vi "TrALEX_GRN.vi"(0 "Analog Amplitude":dbl=1.0 format="%0.2p", 1 "Repetition Frequency":dbl=2.0 format="%.6f") -> ()   [LabVIEW 2011]
uses:
  <vilib>/DAQmx/write.llb/DAQmx Write (Analog Wfm 1Chan NSamp).vi
  <vilib>/DAQmx/create/channels.llb/DAQmx Create Channel (AO-Voltage-Basic).vi
  <vilib>/DAQmx/configure/timing.llb/DAQmx Timing (Sample Clock).vi
  <vilib>/DAQmx/create/channels.llb/DAQmx Create Channel (CO-Pulse Generation-Frequency).vi
  <vilib>/DAQmx/configure/events/hardwareSignals.llb/DAQmx Export Signal (Most Signals).vi
  <vilib>/DAQmx/configure/trigger.llb/DAQmx Start Trigger (Digital Edge).vi
  <vilib>/DAQmx/configure/timing.llb/DAQmx Timing (Implicit).vi
  <vilib>/DAQmx/miscellaneous.llb/DAQmx Fill In Error Info.vi
  <vilib>/measure/NI_MABase.lvlib
panel:
  in  "Three Colour Duty Cycle":dbl=0.3333333333333333 format="%.6f"
  in  "Stop Button":bool
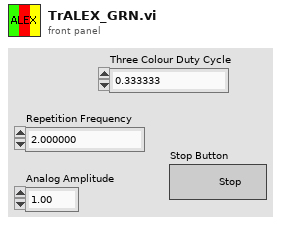
[diagram p1: front panel]
types:
  T1 = enum16{"Sine Wave", "Triangle Wave", "Square Wave", "Sawtooth Wave"}
  T2 = cluster{"Ao0 Sample Clock Rate":dbl, "Ao0 Sample Clock Rate":dbl}
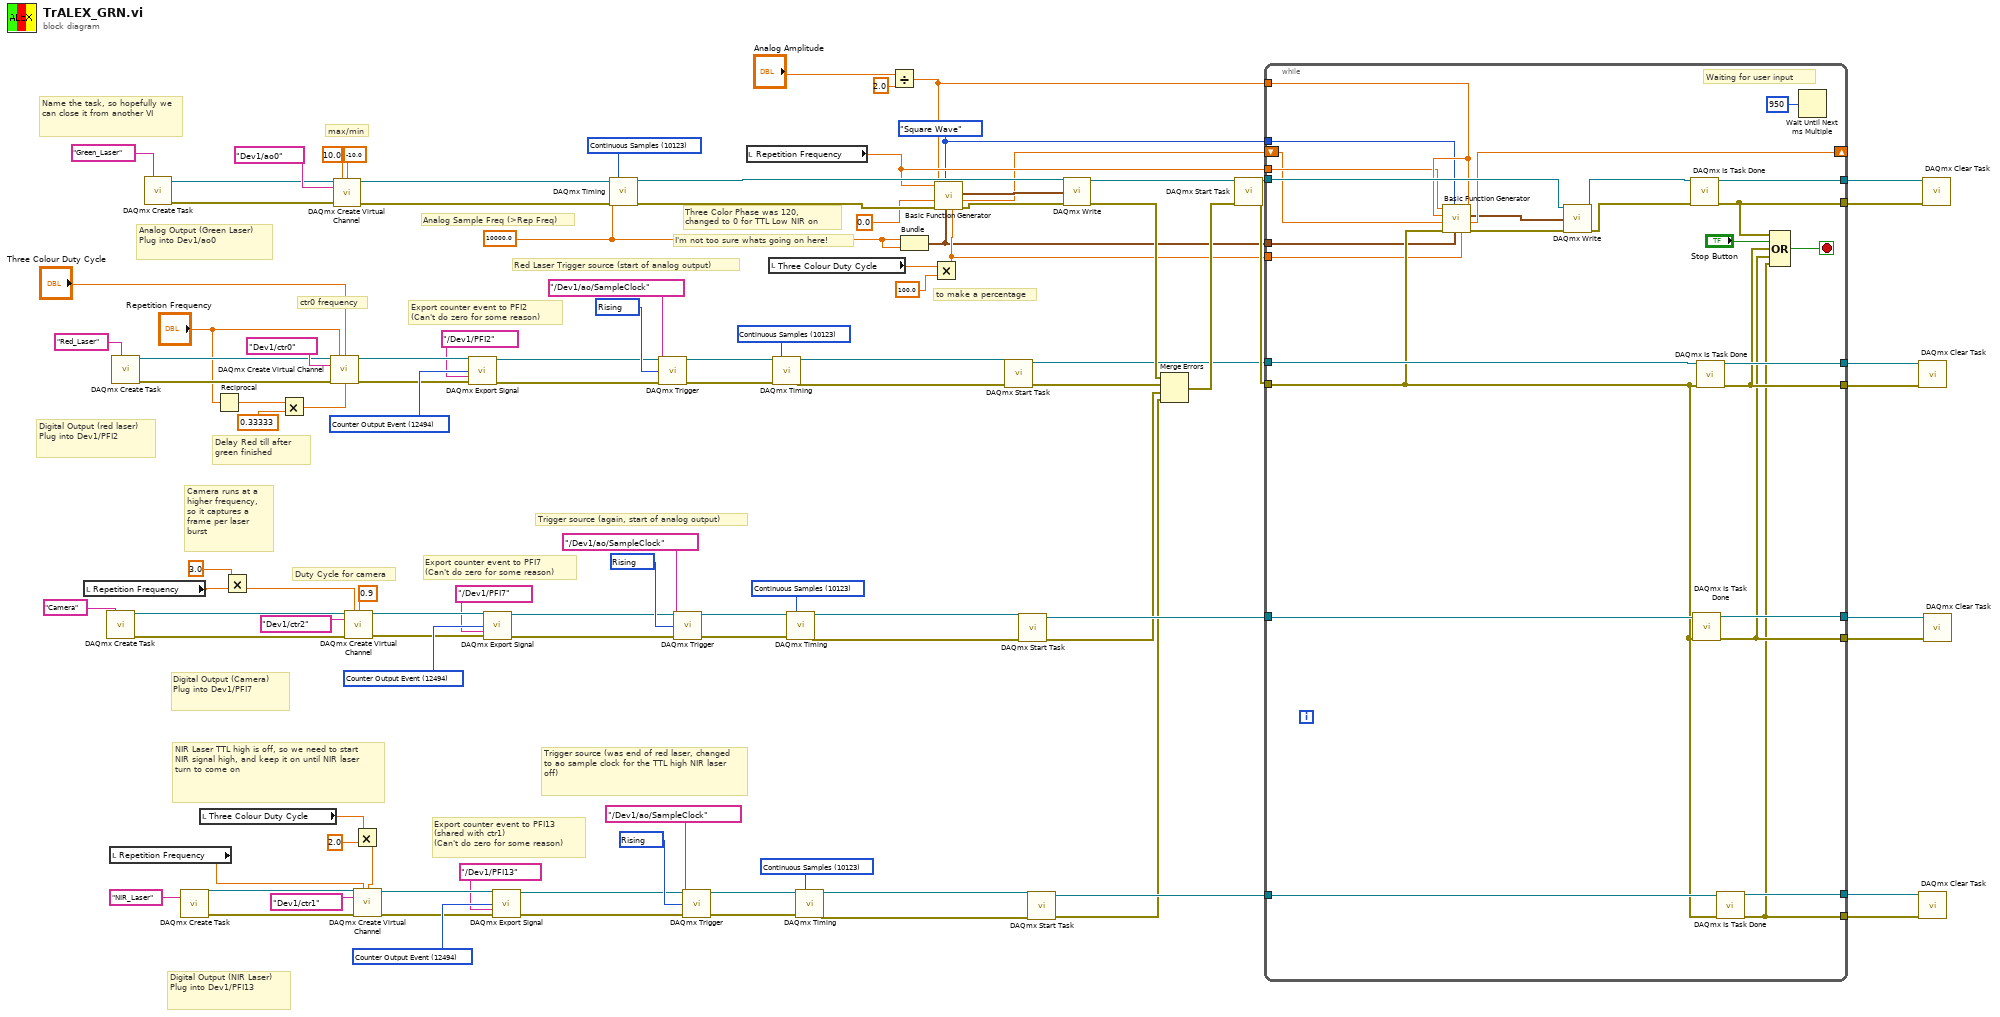
[diagram p0: block diagram]
diagram:
  w41 = 10280 items=["Rising"=10280, "Falling"=10171] ("edge")
  w44 = 10123 items=["Finite Samples"=10178, "Continuous Samples"=10123, "Hardware Timed Single Point"=12522] ("sample mode")
  w46 = 12494 items=["AI Convert Clock"=12484, "10MHz Reference Clock"=12536, "20MHz Timebase Clock"=12486, "Sample Clock"=12487, "Advance Trigger"=12488, "Reference Trigger"=12490, "Start Trigger"=12491, "Advance Complete Event"=12492, "AI Hold Complete Event"=12493, "Counter Output Event"=12494, "Change Detection Event"=12511, "Watchdog Timer Expired Event"=12512] ("signal")
  w64 = 10280 items=["Rising"=10280, "Falling"=10171] ("edge")
  w67 = 10123 items=["Finite Samples"=10178, "Continuous Samples"=10123, "Hardware Timed Single Point"=12522] ("sample mode")
  w69 = 12494 items=["AI Convert Clock"=12484, "10MHz Reference Clock"=12536, "20MHz Timebase Clock"=12486, "Sample Clock"=12487, "Advance Trigger"=12488, "Reference Trigger"=12490, "Start Trigger"=12491, "Advance Complete Event"=12492, "AI Hold Complete Event"=12493, "Counter Output Event"=12494, "Change Detection Event"=12511, "Watchdog Timer Expired Event"=12512] ("signal")
  w75 = 10123 items=["Finite Samples"=10178, "Continuous Samples"=10123, "Hardware Timed Single Point"=12522] ("sample mode")
  w7 = T1."Square Wave" ("signal type")
  w95 = 10280 items=["Rising"=10280, "Falling"=10171] ("edge")
  w100 = 10123 items=["Finite Samples"=10178, "Continuous Samples"=10123, "Hardware Timed Single Point"=12522] ("sample mode")
  w102 = 12494 items=["AI Convert Clock"=12484, "10MHz Reference Clock"=12536, "20MHz Timebase Clock"=12486, "Sample Clock"=12487, "Advance Trigger"=12488, "Reference Trigger"=12490, "Start Trigger"=12491, "Advance Complete Event"=12492, "AI Hold Complete Event"=12493, "Counter Output Event"=12494, "Change Detection Event"=12511, "Watchdog Timer Expired Event"=12512] ("signal")
  w48 = 10000.0 ("Ao0 Sample Clock Rate")
  # "NIR Laser TTL high is off, so we need to start NIR signal high, and keep it on until NIR laser turn to come on"
  # "Delay Red till after green finished"
  # "Name the task, so hopefully we can close it from another VI"
  # "to make a percentage"
  # "Digital Output (NIR Laser) Plug into Dev1/PFI13"
  # "Trigger source (was end of red laser, changed to ao sample clock for the TTL high NIR laser off)"
  # "Export counter event to PFI13 (shared with ctr1)\n(Can't do zero for some reason)"
  # "Duty Cycle for camera"
  # "Camera runs at a higher frequency, so it captures a frame per laser burst"
  # "Digital Output (Camera) Plug into Dev1/PFI7"
  # "Trigger source (again, start of analog output)"
  # "Export counter event to PFI7\n(Can't do zero for some reason)"
  # "Digital Output (red laser) Plug into Dev1/PFI2"
  # "Analog Output (Green Laser) Plug into Dev1/ao0"
  # "Three Color Phase was 120, changed to 0 for TTL Low NIR on"
  # "Analog Sample Freq (>Rep Freq)"
  # "I'm not too sure whats going on here!"
  # "Red Laser Trigger source (start of analog output)"
  # "Export counter event to PFI2\n(Can't do zero for some reason)"
  # "ctr0 frequency"
  # "max/min"
  n1 = local read "Repetition Frequency"() -> (w56:dbl)
  n2 = call <vilib>:"DAQmx Create Task.vi"("new task name"="Camera") -> ("task out"=w16:refnum<k21>, "error out"=w15:errorcluster)  [unwired: 13 in]
  n3 = local read "Repetition Frequency"() -> (w26:dbl)
  n4 = call <vilib>:"DAQmx Create Task.vi"("new task name"="Red_Laser") -> ("task out"=w18:refnum<k21>, "error out"=w17:errorcluster)  [unwired: 13 in]
  n5 = call <vilib>:"DAQmx Create Task.vi"("new task name"="Green_Laser") -> ("task out"=w24:refnum<k21>, "error out"=w23:errorcluster)  [unwired: 13 in]
  n6 = call <vilib>:"DAQmx Create Task.vi"("new task name"="NIR_Laser") -> ("task out"=w14:refnum<k21>, "error out"=w13:errorcluster)  [unwired: 13 in]
  n7 = local read "Three Colour Duty Cycle"() -> (w30:dbl)
  n8 = Reciprocal(x="Repetition Frequency") -> (1/x=w3:dbl)
  n9 = Multiply(x=3.0 ("Repetition Frequency"), y=w56) -> (x*y=w55:dbl)
  n10 = Multiply(x=w3, y=0.33333 ("x")) -> (x*y=w5:dbl)
  n11 = call-poly <vilib>:"DAQmx Create Virtual Channel.vi"("task in"=w18, "frequency"="Repetition Frequency", "duty cycle"="Three Colour Duty Cycle", "counter"=tag "Dev1/ctr0", "error in"=w17, "initial delay"=w5) -> ("task out"=w103:refnum<k21>, "error out"=w101:errorcluster)  [unwired: 8 in]
  n12 = call-poly <vilib>:"DAQmx Create Virtual Channel.vi"("task in"=w24, "maximum value"=10.0, "minimum value"=-10.0, "physical channels"=tag "Dev1/ao0", "error in"=w23) -> ("task out"=w107:refnum<k21>, "error out"=w106:errorcluster)  [unwired: 9 in]
  n13 = call-poly <vilib>:"DAQmx Create Virtual Channel.vi"("task in"=w16, "frequency"=w55, "duty cycle"=0.9, "counter"=tag "Dev1/ctr2", "error in"=w15) -> ("task out"=w70:refnum<k21>, "error out"=w68:errorcluster)  [unwired: 9 in]
  n14 = Multiply(x=w30, y=2.0) -> (x*y=w2:dbl)
  n15 = call-poly <vilib>:"DAQmx Create Virtual Channel.vi"("task in"=w14, "frequency"=w26, "duty cycle"=w2, "counter"=tag "Dev1/ctr1", "error in"=w13) -> ("task out"=w47:refnum<k21>, "error out"=w45:errorcluster)  [unwired: 9 in]
  n16 = call-poly <vilib>:"DAQmx Export Signal.vi"("task/channels in"=w103, "signal"=w102, "output terminal"=tag "/Dev1/PFI2", "error in"=w101) -> ("task out"=w94:refnum<k21>, "error out"=w91:errorcluster)  [unwired: 10 in]
  n17 = call-poly <vilib>:"DAQmx Export Signal.vi"("task/channels in"=w70, "signal"=w69, "output terminal"=tag "/Dev1/PFI7", "error in"=w68) -> ("task out"=w63:refnum<k21>, "error out"=w60:errorcluster)  [unwired: 10 in]
  n18 = call-poly <vilib>:"DAQmx Export Signal.vi"("task/channels in"=w47, "signal"=w46, "output terminal"=tag "/Dev1/PFI13", "error in"=w45) -> ("task out"=w40:refnum<k21>, "error out"=w37:errorcluster)  [unwired: 10 in]
  n19 = call-poly <vilib>:"DAQmx Timing.vi"("task/channels in"=w107, "sample mode"=w75, "rate"=w48, "error in"=w106) -> ("task out"=w99:refnum<k21>, "error out"=w98:errorcluster)  [unwired: 10 in]
  n20 = call-poly <vilib>:"DAQmx Trigger.vi"("task/channels in"=w94, "source"=tag "/Dev1/ao/SampleClock", "edge"=w95, "error in"=w91) -> ("task out"=w93:refnum<k21>, "error out"=w92:errorcluster)  [unwired: 10 in]
  n21 = call-poly <vilib>:"DAQmx Trigger.vi"("task/channels in"=w63, "source"=tag "/Dev1/ao/SampleClock", "edge"=w64, "error in"=w60) -> ("task out"=w62:refnum<k21>, "error out"=w61:errorcluster)  [unwired: 10 in]
  n22 = call-poly <vilib>:"DAQmx Trigger.vi"("task/channels in"=w40, "source"=tag "/Dev1/ao/SampleClock", "edge"=w41, "error in"=w37) -> ("task out"=w39:refnum<k21>, "error out"=w38:errorcluster)  [unwired: 10 in]
  n23 = local read "Repetition Frequency"() -> (w12:dbl)
  n24 = local read "Three Colour Duty Cycle"() -> (w32:dbl)
  n25 = call-poly <vilib>:"DAQmx Timing.vi"("task/channels in"=w93, "sample mode"=w100, "error in"=w92) -> ("task out"=w88:refnum<k21>, "error out"=w87:errorcluster)  [unwired: 11 in]
  n26 = call-poly <vilib>:"DAQmx Timing.vi"("task/channels in"=w62, "sample mode"=w67, "error in"=w61) -> ("task out"=w59:refnum<k21>, "error out"=w58:errorcluster)  [unwired: 11 in]
  n27 = call-poly <vilib>:"DAQmx Timing.vi"("task/channels in"=w39, "sample mode"=w44, "error in"=w38) -> ("task out"=w36:refnum<k21>, "error out"=w35:errorcluster)  [unwired: 11 in]
  n28 = Divide(x="Analog Amplitude", y=2.0) -> (x/y=w11:dbl)
  n29 = Bundle("Ao0 Sample Clock Rate"=w48, "Ao0 Sample Clock Rate"=w48) -> (w8:T2)  [unwired: 1 in]
  n30 = Multiply(x=w32, y=100.0) -> (x*y=w9:dbl)
  n31 = call <vilib>:"Basic Function Generator.vi"("offset"=w11, "square wave duty cycle (%)"=w9, "sampling info"=w8, "signal type"=w7, "error in (no error)"=w98, "phase"=0.0, "amplitude"=w11, "frequency"=w12) -> ("error out"=w89:errorcluster, "phase out"=w10:dbl, "signal out"=w90:waveform(dbl))  [unwired: 1 in]
  n32 = call <vilib>:"DAQmx Start Task.vi"("task/channels in"=w88, "error in"=w87) -> ("task out"=w76:refnum<k21>, "error out"=w86:errorcluster)  [unwired: 12 in]
  n33 = call <vilib>:"DAQmx Start Task.vi"("task/channels in"=w59, "error in"=w58) -> ("task out"=w52:refnum<k21>, "error out"=w51:errorcluster)  [unwired: 12 in]
  n34 = call <vilib>:"DAQmx Start Task.vi"("task/channels in"=w36, "error in"=w35) -> ("task out"=w29:refnum<k21>, "error out"=w25:errorcluster)  [unwired: 12 in]
  n35 = call-poly <vilib>:"DAQmx Write.vi"("task/channels in"=w99, "data"=w90, "error in"=w89) -> ("task out"=w83:refnum<k21>, "error out"=w85:errorcluster)  [unwired: 10 in, 1 out]
  n36 = Merge Errors(w85, w86, w51, w25) -> (w84:errorcluster)
  n37 = call <vilib>:"DAQmx Start Task.vi"("task/channels in"=w83, "error in"=w84) -> ("task out"=w82:refnum<k21>, "error out"=w81:errorcluster)  [unwired: 12 in]
  n38 = while {
    tunnel: [w135] -> w77
    tunnel: [w129] -> w80
    tunnel: [w132] -> w78
    tunnel: [w127] -> w79
    tunnel: w82 -> [w117]
    tunnel: w81 -> [w121]
    tunnel: w76 -> [w131]
    tunnel: w52 -> [w130]
    tunnel: [w126] -> w50
    tunnel: [w125] -> w49
    tunnel: w29 -> [w124]
    tunnel: [w123] -> w28
    tunnel: [w122] -> w27
    tunnel: w12 -> [w115]
    tunnel: w11 -> [w116]
    shift-right: [w113] -> _
    shift-left: w10 -> [w114]
    tunnel: w9 -> [w111]
    tunnel: w8 -> [w110]
    tunnel: w7 -> [w109]
    stop <- w133 stop-if-true
    # "Waiting for user input"
    n39 = call <vilib>:"Basic Function Generator.vi"("offset"=w116, "square wave duty cycle (%)"=w111, "sampling info"=w110, "signal type"=w109, "error in (no error)"=w121, "phase"=w114, "amplitude"=w116, "frequency"=w115) -> ("error out"=w120:errorcluster, "phase out"=w113:dbl, "signal out"=w112:waveform(dbl))  [unwired: 1 in]
    n40 = call-poly <vilib>:"DAQmx Write.vi"("task/channels in"=w117, "data"=w112, "error in"=w120) -> ("task out"=w118:refnum<k21>, "error out"=w119:errorcluster)  [unwired: 10 in, 1 out]
    n41 = call <vilib>:"DAQmx Is Task Done.vi"("task/channels in"=w118, "error in"=w119) -> ("task out"=w135:refnum<k21>, "error out"=w129:errorcluster)  [unwired: 11 in, 1 out]
    n42 = call <vilib>:"DAQmx Is Task Done.vi"("task/channels in"=w130, "error in"=w121) -> ("task out"=w126:refnum<k21>, "error out"=w125:errorcluster)  [unwired: 11 in, 1 out]
    n43 = call <vilib>:"DAQmx Is Task Done.vi"("task/channels in"=w131, "error in"=w121) -> ("task out"=w132:refnum<k21>, "error out"=w127:errorcluster)  [unwired: 11 in, 1 out]
    n44 = call <vilib>:"DAQmx Is Task Done.vi"("task/channels in"=w124, "error in"=w121) -> ("task out"=w123:refnum<k21>, "error out"=w122:errorcluster)  [unwired: 11 in, 1 out]
    n45 = Compound Arithmetic op=OR(w129, "Stop Button", w127, w125, w122) -> (w133:bool)
    n46 = Wait Until Next ms Multiple(millisecond multiple=u32 950) -> ()  [unwired: 1 out]
  }
  n47 = call <vilib>:"DAQmx Clear Task.vi"("task in"=w78, "error in"=w79) -> ()  [unwired: 13 in, 1 out]
  n48 = call <vilib>:"DAQmx Clear Task.vi"("task in"=w28, "error in"=w27) -> ()  [unwired: 13 in, 1 out]
  n49 = call <vilib>:"DAQmx Clear Task.vi"("task in"=w77, "error in"=w80) -> ()  [unwired: 13 in, 1 out]
  n50 = call <vilib>:"DAQmx Clear Task.vi"("task in"=w50, "error in"=w49) -> ()  [unwired: 13 in, 1 out]
